vi "PH_Strings.convert Time 1.vi"(1 "Date":string, 2 "Time":string) -> (0 "Time":timestamp)   [LabVIEW 2014, in "PH_Common.lvlib"]
doc: "This VI converts a LabVIEW Time and Date string to a LabVIEW timestamp."
uses:
  PH_Common.lvlib
panel:
  in  "date time rec":T1
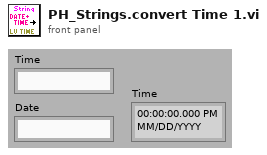
[diagram p1: front panel]
types:
  T1 = cluster{"second":i32, "minute":i32, "hour":i32, "day of month":i32, "month":i32, "year":i32, "day of week":i32, "day of year":i32, "is DST":i32}
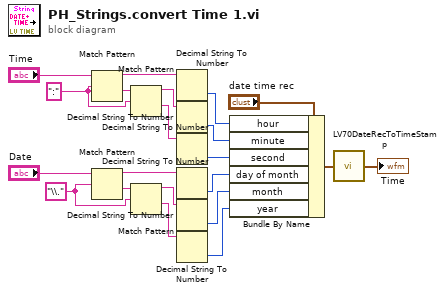
[diagram p0: block diagram]
diagram:
  w21 = "\\." ("regular expression")
  w5 = ":" ("regular expression")
  n1 = Match Pattern(string="Time", regular expression=w5) -> (before substring=w6:string, after substring=w4:string)  [unwired: 1 in, 2 out]
  n2 = Match Pattern(string="Date", regular expression=w21) -> (before substring=w14:string, after substring=w13:string)  [unwired: 1 in, 2 out]
  n3 = Match Pattern(string=w4, regular expression=w5) -> (before substring=w7:string, after substring=w8:string)  [unwired: 1 in, 2 out]
  n4 = Match Pattern(string=w13, regular expression=w21) -> (before substring=w15:string, after substring=w16:string)  [unwired: 1 in, 2 out]
  n5 = Decimal String To Number(string=w6) -> (number=w10:i32)  [unwired: 2 in, 1 out]
  n6 = Decimal String To Number(string=w7) -> (number=w11:i32)  [unwired: 2 in, 1 out]
  n7 = Decimal String To Number(string=w8) -> (number=w12:i32)  [unwired: 2 in, 1 out]
  n8 = Decimal String To Number(string=w14) -> (number=w17:i32)  [unwired: 2 in, 1 out]
  n9 = Decimal String To Number(string=w15) -> (number=w18:i32)  [unwired: 2 in, 1 out]
  n10 = Decimal String To Number(string=w16) -> (number=w19:i32)  [unwired: 2 in, 1 out]
  n11 = Bundle By Name(cluster="date time rec", "hour"=w10, "minute"=w11, "second"=w12, "day of month"=w17, "month"=w18, "year"=w19) -> (w20:T1)
  n12 = call <vilib>:"LV70DateRecToTimeStamp.vi"("date time rec"=w20) -> ("Time Stamp"=→"Time":timestamp)
